vi "get system version.vi"(8 "error in (no error)":errorcluster, 11 "engine in":refnum<class "Engine Parent Editor Node.lvclass">) -> (0 "error out":errorcluster, 2 "version":T1, 3 "engine out":refnum<class "Engine Parent Editor Node.lvclass">)   [LabVIEW 2014, in "Shared Memory editor node.lvclass"]
uses:
  Shared Memory editor node.lvclass
  <vilib>/NI/DCAF/Tag Editor Core/Configuration Editor/Classes/Engine Parent/Engine Parent Editor Node.lvclass
  <vilib>/NI/Configuration Framework/Node/NISE_CEF_Node.lvclass/NISE_CEF_Node.ctl
  <vilib>/NI/DCAF/Tag Editor Core/Configuration Editor/Classes/Systems/Systems.lvclass
  <vilib>/NI/Configuration Framework/Node/ReadParent.vi
  <vilib>/NI/Configuration Framework/Node/NISE_CEF_Node.lvclass
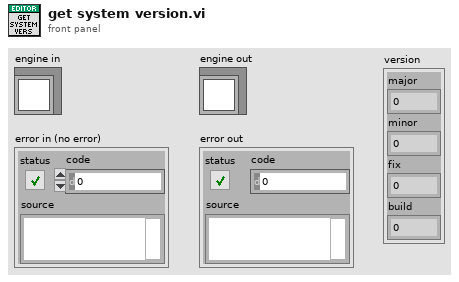
[diagram p1: front panel]
types:
  T1 = cluster{"major":u16, "minor":u16, "fix":u16, "build":u16}
  T2 = typedef "NISE_CEF_Node.lvclass/NodeRef.ctl" = refnum<data-value>
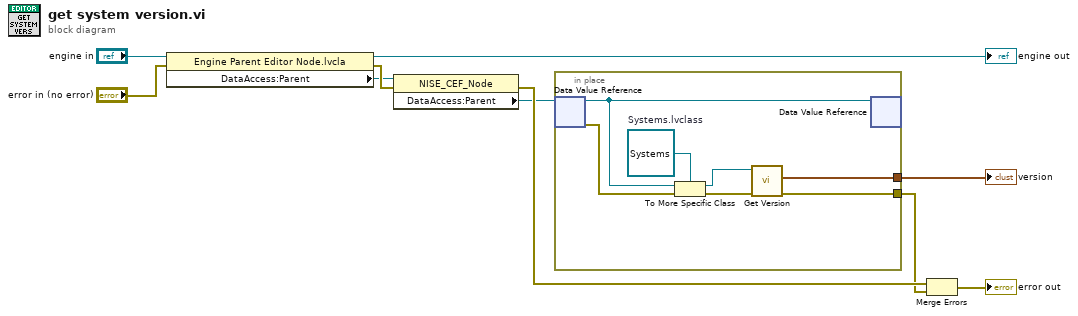
[diagram p0: block diagram]
diagram:
  n1 = property class="Engine Parent Editor Node.lvcla"(reference="engine in", error in="error in (no error)") -> (reference out=→"engine out":refnum<class "Engine Parent Editor Node.lvclass">, error out=w8:errorcluster, "DataAccess:Parent"=w4:T2)
  n2 = property class="NISE_CEF_Node"(reference=w4, error in=w8) -> (error out=w9:errorcluster, "DataAccess:Parent"=w3:T2)  [unwired: 1 out]
  n3 = in-place {
    in-place-border: [w12] -> w2
    in-place-border: [w11] -> w1
    w17 = refnum<class "Systems.lvclass"> refnum  # Systems.lvclass
    n4 = in-place-dvr #1(w3) -> (w15:refnum<class "NISE_CEF_Node.lvclass">, w16:errorcluster)
    n5 = To More Specific Class(target class=w17, reference=w15, error in=w16) -> (specific class reference=w13:refnum<class "Systems.lvclass">, error out=w14:errorcluster)
    n6 = call <vilib>:"Get Version.vi"("error in (no error)"=w14, "system in"=w13) -> ("error out"=w12:errorcluster, "version"=w11:T1)  [unwired: 7 in, 1 out]
    n7 = in-place-dvr #1(w15) -> ()  [unwired: 2 out]
  }
  "version" <- w1
  n8 = Merge Errors(w9, w2) -> (→"error out":errorcluster)
